vi "Set_Range.vi"(0 "VisaCluster":T2, 7 "Range":T1, 11 "error in (no error)":errorcluster) -> (4 "VisaCluster":T2, 6 "Range":T1, 8 "Answer":string, 15 "error out":errorcluster)   [LabVIEW 2014, in "FH 55.lvlib"]
doc: "This VI sets the Range on 1, 2, 3, 4, 5, 6, 7.\n\n1 = 30 mikro Tesla, 2 = 300 mikro Tesla, 3 = 3 mili Tesla, 4 = 30 mili Tesla, 5 = 300 mili Tesla, 6 = 3 Tesla, 7 = 30 Telar. \n\nDurch das VI kann der Messbereich manuell gewählt werden. Welche Messbereiche vorhanden sind, hängt von der Sonde ab, so dass einige Bereiche eine Fehlermeldung erzeugen können."
uses:
  FH 55.lvlib
  TypeDef/VisaCluster.ctl
  TypeDef/Range.ctl
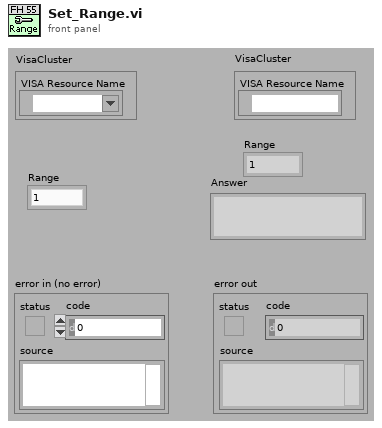
[diagram p1: front panel]
types:
  T1 = typedef "FH 55.lvlib/Range.ctl" = enum16{"1", "2", "3", "4", "5", "6", "7"}
  T2 = typedef "FH 55.lvlib/VisaCluster.ctl" = cluster{"VISA Resource Name":refnum<visa-resource-name>}
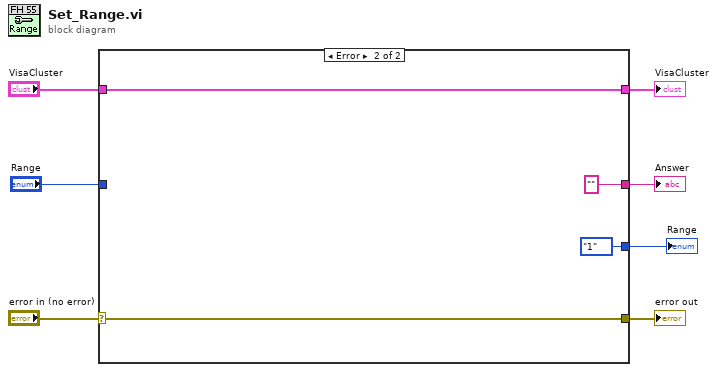
[diagram p0: block diagram]
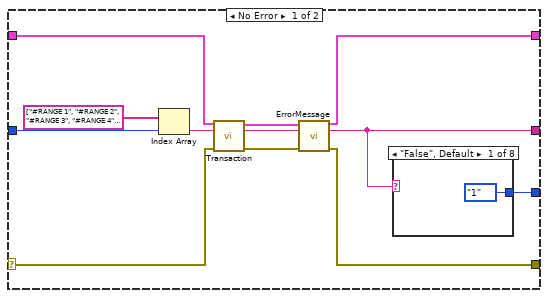
[diagram p2: hidden frame]
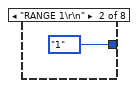
[diagram p3: hidden frame]
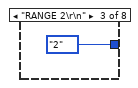
[diagram p4: hidden frame]
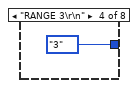
[diagram p5: hidden frame]
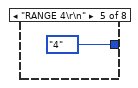
[diagram p6: hidden frame]
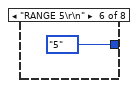
[diagram p7: hidden frame]
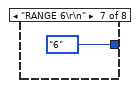
[diagram p8: hidden frame]
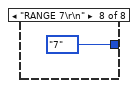
[diagram p9: hidden frame]
diagram:
  n1 = case shown="Error" "error in (no error)" {
    selector: "error in (no error)" -> [w16 w30]
    tunnel: "VisaCluster" -> [w17 w31]
    tunnel: "Range" -> [w12 _]
    tunnel: [w19 w31] -> w3
    tunnel: [w18 w30] -> w5
    tunnel: [w9 ""] -> w4
    tunnel: [w8 Range."1" ("Range")] -> w1
    frame No Error {
      n2 = Index Array(array=string[] ["#RANGE 1", "#RANGE 2", "#RANGE 3", "#RANGE 4", "#RANGE 5", "#RANGE 6", "#RANGE 7", ""], index=w12) -> (element=w10:string)
      n3 = call "Transaction.vi"("VisaCluster"=w17, "Command"=w10, "error in (no error)"=w16) -> ("VisaCluster"=w13:T2, "Answer"=w14:string, "error out"=w15:errorcluster)  [unwired: 9 in, 1 out]
      n4 = call "ErrorMessage.vi"("VisaCluster"=w13, "Message In"=w14, "error in (no error)"=w15) -> ("VisaCluster"=w19:T2, "Message Out"=w9:string, "error out"=w18:errorcluster)  [unwired: 10 in]
      n5 = case shown="\"False\", Default" w9 {
        tunnel: [Range."1" ("Range") Range."1" ("Range") Range."2" ("Range") Range."3" ("Range") Range."4" ("Range") Range."5" ("Range") Range."6" ("Range") Range."7" ("Range")] -> w8
        frame "False", Default {
        }
        frame "RANGE 1\r\n" {
        }
        frame "RANGE 2\r\n" {
        }
        frame "RANGE 3\r\n" {
        }
        frame "RANGE 4\r\n" {
        }
        frame "RANGE 5\r\n" {
        }
        frame "RANGE 6\r\n" {
        }
        frame "RANGE 7\r\n" {
        }
      }
    }
    frame Error {
    }
  }
  "error out" <- w5
  "Answer" <- w4
  "VisaCluster" <- w3
  "Range" <- w1
